vi "Save to Spreadsheet file.vi"(6 "Version (Excel 2007+)":enum16{"Excel 2007+", "Excel 2003-"}(ring), 7 "sheetname":string="Sheet1", 8 "error in (no error)":errorcluster, 10 "Values":string[][](array[string]), 11 "File Name":path=path "C:/PhaeronGit/LVNPOI/Scratch/test.xls") -> (0 "error out":errorcluster)   [LabVIEW 2013]
doc: "Writes the 2D string array to the named Excel format file."
uses:
  OOP/Spreadsheet.lvclass
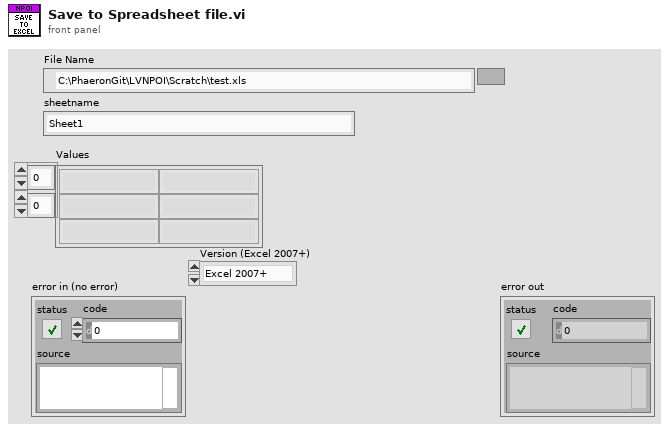
[diagram p1: front panel]
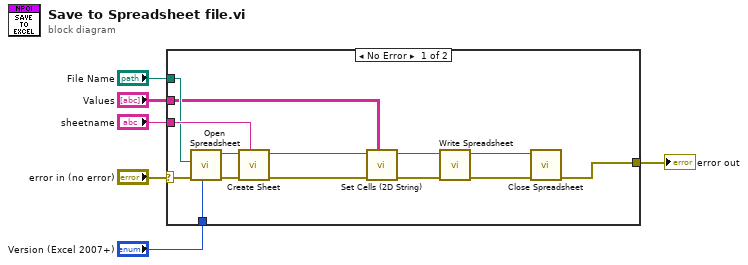
[diagram p0: block diagram]
diagram:
  n1 = case shown="No Error" "error in (no error)" {
    selector: "error in (no error)" -> [w20 w21]
    tunnel: "File Name" -> [w14 _]
    tunnel: "sheetname" -> [w16 _]
    tunnel: [w15 w21] -> w4
    tunnel: "Values" -> [w7 _]
    tunnel: "Version (Excel 2007+)" -> [w19 _]
    frame No Error {
      n2 = call "Open Spreadsheet.vi"("Version (Excel 2007+)"=w19, "error in (no error)"=w20, "File Name"=w14) -> ("error out"=w18:errorcluster, "Spreadsheet"=w17:refnum<class "Spreadsheet.lvclass">)  [unwired: 7 in]
      n3 = call-dynamic "Create Sheet.vi"("Sheet Name (Sheet1)"=w16, "error in (no error)"=w18, "Spreadsheet in"=w17) -> ("error out"=w9:errorcluster, "Spreadsheet out"=w11:refnum<class "Spreadsheet.lvclass">)  [unwired: 7 in]
      n4 = call-dynamic "Set Cells (2D String).vi"("Values"=w7, "error in (no error)"=w9, "Spreadsheet in"=w11) -> ("error out"=w8:errorcluster, "Spreadsheet out"=w10:refnum<class "Spreadsheet.lvclass">)  [unwired: 7 in]
      n5 = call-dynamic "Write Spreadsheet.vi"("error in (no error)"=w8, "Spreadsheet in"=w10) -> ("error out"=w13:errorcluster, "Spreadsheet out"=w12:refnum<class "Spreadsheet.lvclass">)  [unwired: 8 in]
      n6 = call-dynamic "Close Spreadsheet.vi"("error in (no error)"=w13, "Spreadsheet in"=w12) -> ("error out"=w15:errorcluster)  [unwired: 8 in, 1 out]
    }
    frame Error {
    }
  }
  "error out" <- w4
